vi "Init Wfm Capture.vi"(8 "error in (no error)":errorcluster, 11 "Actor_Scope in":refnum<class "Actor_Scope.lvclass">) -> (0 "error out":errorcluster, 3 "Actor_Scope out":refnum<class "Actor_Scope.lvclass">)   [LabVIEW 2020, in "Actor_Scope.lvlib" / "Actor_Scope.lvclass"]
uses:
  Actor_Scope.lvclass
  C:/Program Files/National Instruments/LabVIEW 2020/vi.lib/ActorFramework/Actor/Actor.lvclass
  Scope_Event.ctl
  <vilib>/ActorFramework/Actor/Actor.lvclass/Actor.ctl
  Actor_Scope.lvclass/Actor_Scope.ctl
  <instrlib>/Agilent 8000 Series/Agilent 8000 Series.lvlib
  <vilib>/ActorFramework/Actor/Actor.lvclass
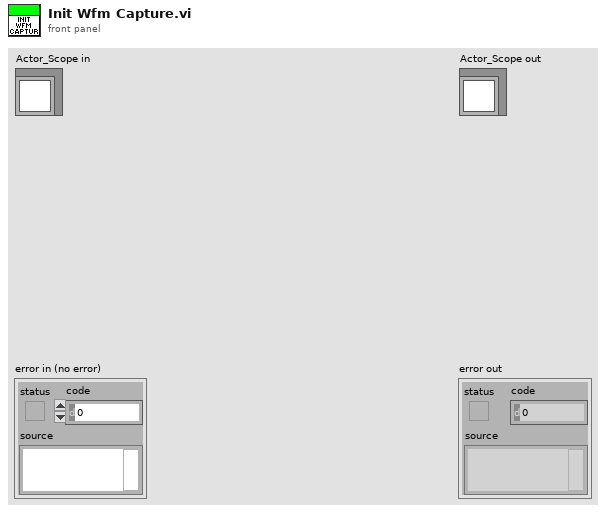
[diagram p1: front panel]
types:
  T1 = typedef "Actor_Scope.lvlib/Actor_Scope.lvclass/Scope_Event.ctl" = enum16{"General Event", "Inited", "Error", "Res Read complete", "Wfm Acq Complete"}
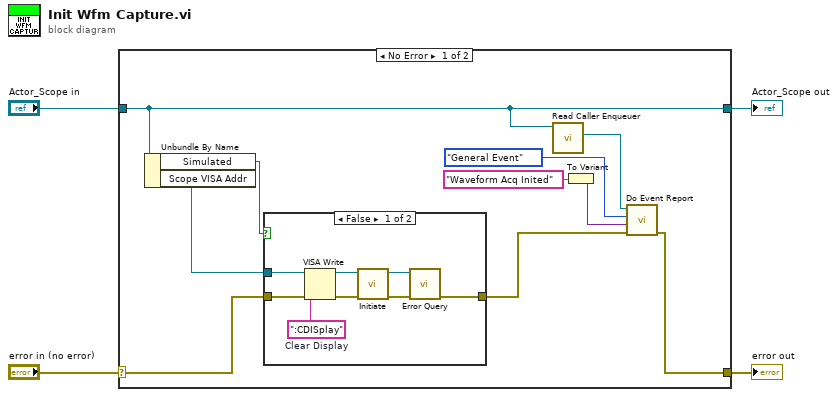
[diagram p0: block diagram]
diagram:
  n1 = case shown="No Error" "error in (no error)" {
    selector: "error in (no error)" -> [w6 w25]
    tunnel: [w8 w25] -> w3
    tunnel: [w13 w24] -> w1
    tunnel: "Actor_Scope in" -> [w13 w24]
    frame No Error {
      n2 = Unbundle By Name(w13) -> ("Simulated"=w5:bool, "Scope VISA Addr"=w7:refnum<visa-resource-name>)
      n3 = case shown="False" w5 {
        tunnel: [w20 w23] -> w9
        tunnel: w7 -> [w19 _]
        tunnel: w6 -> [w18 w23]
        frame False {
          w17 = ":CDISplay"  # Clear Display
          n4 = VISA Write(VISA resource name=w19, write buffer=w17, error in (no error)=w18) -> (VISA resource name out=w16:refnum<visa-resource-name>, error out=w15:errorcluster)  [unwired: 1 out]
          n5 = call <instrlib>:"Initiate.vi"("error in (no error)"=w15, "VISA resource name"=w16) -> ("error out"=w21:errorcluster, "VISA resource name out"=w22:refnum<visa-resource-name>)  [unwired: 8 in]
          n6 = call <instrlib>:"Error Query.vi"("error in (no error)"=w21, "VISA resource name"=w22) -> ("error out"=w20:errorcluster)  [unwired: 6 in, 3 out]
        }
        frame True {
        }
      }
      n7 = call <vilib>:"Read Caller Enqueuer.vi"("Actor"=w13) -> ("Caller Enqueuer"=w12:refnum<class "Message Enqueuer.lvclass">)  [unwired: 10 in]
      n8 = To Variant(anything="Waveform Acq Inited") -> (Variant=w10:variant)
      n9 = call "Do Event Report.vi"("error in (no error)"=w9, "Event Data"=w10, "Scope Events"=Scope_Event."General Event", "Caller Enqueuer"=w12) -> ("error out"=w8:errorcluster)  [unwired: 6 in, 1 out]
    }
    frame Error {
    }
  }
  "error out" <- w3
  "Actor_Scope out" <- w1
